vi "dataacq3.vi"() -> ()   [LabVIEW 2014]
uses:
  <vilib>/DAQmx/create/channels.llb/DAQmx Create Channel (AI-Voltage-Basic).vi
  <vilib>/DAQmx/read.llb/DAQmx Read (Analog 2D DBL NChan NSamp).vi
  <vilib>/measure/maspectr.llb/FFT Power Spectrum and PSD for 1 Chan.vi
  <vilib>/DAQmx/create/channels.llb/DAQmx Create Channel (AO-Voltage-Basic).vi
  <vilib>/DAQmx/write.llb/DAQmx Write (Analog 2D DBL NChan NSamp).vi
  <vilib>/measure/NI_MABase.lvlib
  <vilib>/measure/NI_MAPro.lvlib
panel:
  out "Power Spectrum 2":cluster{"f0":dbl, "df":dbl, "magnitude":dbl[]}(graph)
  out "Power Spectrum1":cluster{"f0":dbl, "df":dbl, "magnitude":dbl[]}(graph)
  out "Waveform Chart 2":dbl[][](graph)
  out "error out 2":errorcluster
  in  "Input channels":tag
  in  "stop":bool
  in  "sampling info 2":cluster{"Fs":dbl, "#s":dbl}={"Fs"=1000.0, "#s"=1000.0} {"Fs" format="%.2p"}
  in  "sampling info":cluster{"Fs":dbl, "#s":dbl}={"Fs"=1000.0, "#s"=1000.0} {"Fs" format="%.2p"}
  in  "Phase 2":dbl format="%.2f"
  in  "amplitude 2":dbl=5.0 format="%.2f"
  in  "frequency 2":dbl=1000.0 format="%.2f"
  out "Waveform Chart":dynamicdata(graph)
  in  "Phase":dbl format="%.2f"
  in  "amplitude":dbl=5.0 format="%.2f"
  in  "frequency":dbl=1000.0 format="%.2f"
  in  "output channels":tag
  out "error out":errorcluster
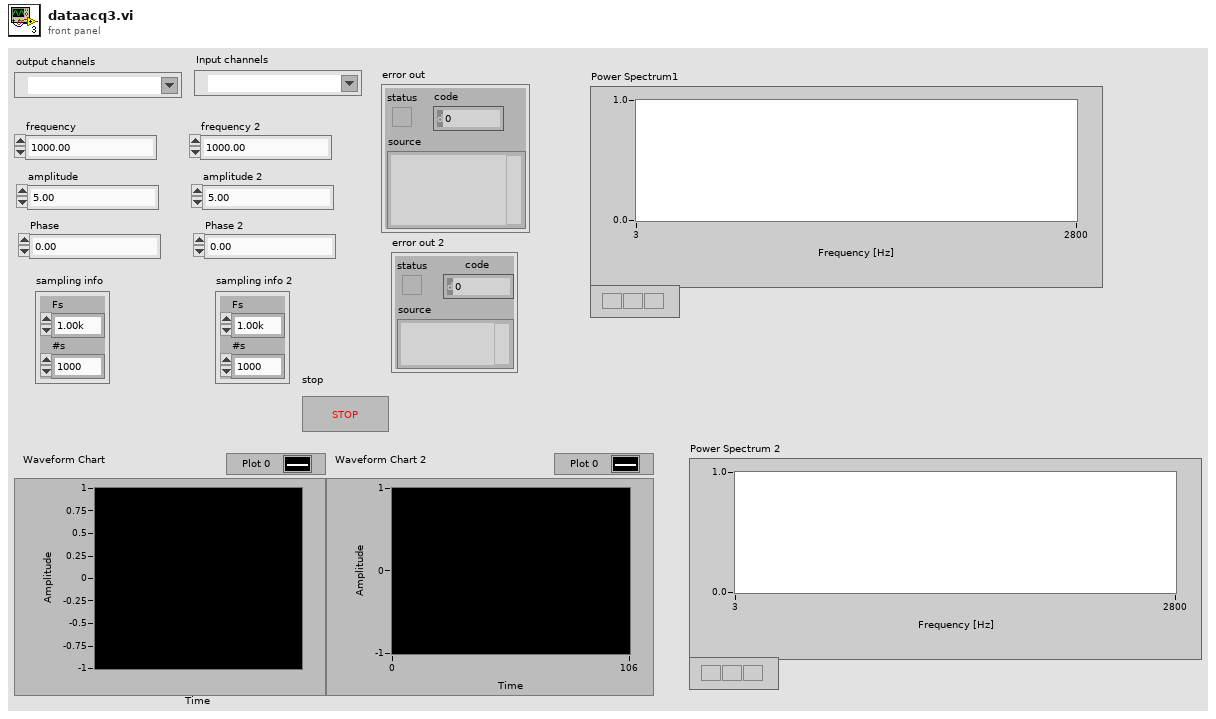
[diagram p1: front panel]
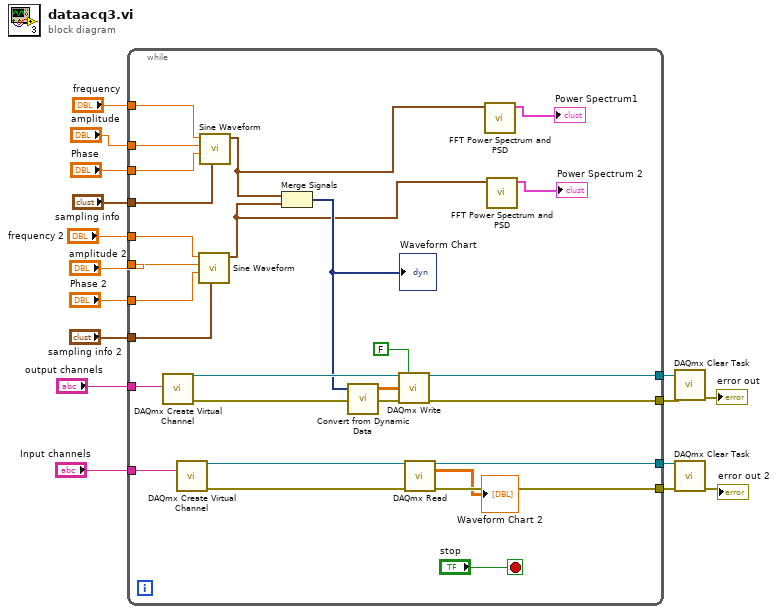
[diagram p0: block diagram]
diagram:
  n1 = while {
    tunnel: [w43] -> w16
    tunnel: [w42] -> w15
    tunnel: "output channels" -> [w41]
    tunnel: "frequency" -> [w40]
    tunnel: "amplitude" -> [w39]
    tunnel: "Phase" -> [w38]
    tunnel: "frequency 2" -> [w36]
    tunnel: "amplitude 2" -> [w35]
    tunnel: "Phase 2" -> [w34]
    tunnel: "sampling info" -> [w33]
    tunnel: "sampling info 2" -> [w32]
    tunnel: "Input channels" -> [w25]
    tunnel: [w24] -> w3
    tunnel: [w23] -> w2
    stop <- "stop" stop-if-true
    n2 = call-poly <vilib>:"DAQmx Create Virtual Channel.vi"("physical channels"=w41) -> ("task out"=w29:refnum<k21>, "error out"=w28:errorcluster)  [unwired: 13 in]
    n3 = call-poly <vilib>:"DAQmx Create Virtual Channel.vi"("physical channels"=w25) -> ("task out"=w27:refnum<k21>, "error out"=w26:errorcluster)  [unwired: 13 in]
    n4 = call <vilib>:"Sine Waveform.vi"("sampling info"=w32, "phase"=w34, "amplitude"=w35, "frequency"=w36) -> ("signal out"=w17:waveform(dbl))  [unwired: 6 in, 1 out]
    n5 = call <vilib>:"Sine Waveform.vi"("sampling info"=w33, "phase"=w38, "amplitude"=w39, "frequency"=w40) -> ("signal out"=w20:waveform(dbl))  [unwired: 6 in, 1 out]
    n6 = Merge Signals(w20, w17) -> (w21:dynamicdata)
    "Waveform Chart" <- w21
    n7 = call "Convert from Dynamic Data"("Dynamic Data Type"=w21) -> ("Array"=w31:dbl[][])  [unwired: 3 in]
    n8 = call-poly <vilib>:"DAQmx Write.vi"("task/channels in"=w29, "auto start"=FALSE, "data"=w31, "error in"=w28) -> ("task out"=w43:refnum<k21>, "error out"=w42:errorcluster)  [unwired: 9 in, 1 out]
    n9 = call-poly <vilib>:"DAQmx Read.vi"("task/channels in"=w27, "error in"=w26) -> ("task out"=w24:refnum<k21>, "data"=→"Waveform Chart 2":dbl[][], "error out"=w23:errorcluster)  [unwired: 11 in]
    n10 = call-poly <vilib>:"FFT Power Spectrum and PSD.vi"("time signal"=w20) -> ("Power Spectrum / PSD"=→"Power Spectrum1":cluster{"f0":dbl, "df":dbl, "magnitude":dbl[]})  [unwired: 7 in, 3 out]
    n11 = call-poly <vilib>:"FFT Power Spectrum and PSD.vi"("time signal"=w17) -> ("Power Spectrum / PSD"=→"Power Spectrum 2":cluster{"f0":dbl, "df":dbl, "magnitude":dbl[]})  [unwired: 7 in, 3 out]
  }
  n12 = call <vilib>:"DAQmx Clear Task.vi"("task in"=w16, "error in"=w15) -> ("error out"=→"error out":errorcluster)  [unwired: 13 in]
  n13 = call <vilib>:"DAQmx Clear Task.vi"("task in"=w3, "error in"=w2) -> ("error out"=→"error out 2":errorcluster)  [unwired: 13 in]
